vi "1ZZTEMPZZ.vi"(8 "error in":errorcluster, 9 "Message":string="Labview Stopped due to Insuficient Space", 10 "Subject":string="Labview Stopped due to Insuficient Space", 11 "Recipients":string="jtp246@cornell.edu") -> (0 "error out":errorcluster)   [LabVIEW 2023]
doc: "<p>Creates and sends an email according to the settings you specify in the configuration dialog box.</p>\n--------------------\n\nThis Express VI is configured as follows:\n\nThis VI can be used to programmatically send emails"
uses:
  GUI2.vi
  <vilib>/smtpClient/LabVIEWSMTPClient.lvlib
panel:
  in  "Require Log-in":bool=TRUE
  in  "Sender's Email Address":string="jtp246@cornell.edu"
  in  "Use Secure Connection (TLS\\SSL":bool=TRUE
  in  "Password":string="yult ybhd eril bmmg"
  in  "Port":u16=25
  in  "Username":string="b56ainvertedmicroscope@gmail.com"
  in  "Outgoing Mail Server (SMTP)":string="smtp.gmail.com"
  # "Refer to the LabVIEW Help,\navailable by selecting\nHelp>Search the\nLabVIEW Help, for\ninformation about\ndesigning \"source VIs\".\n(Include quotes)"
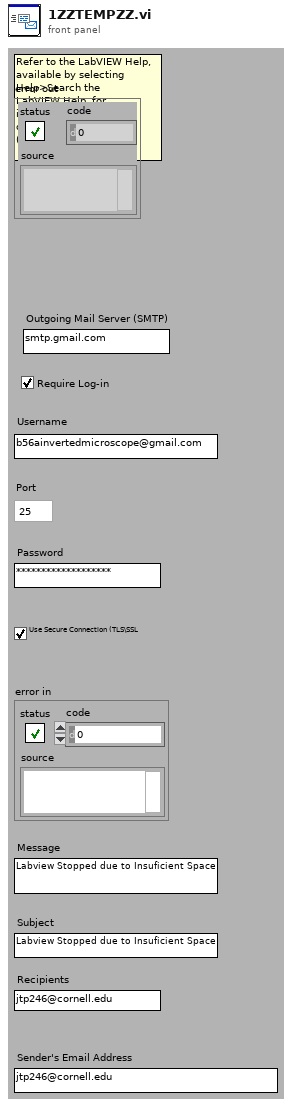
[diagram p1: front panel]
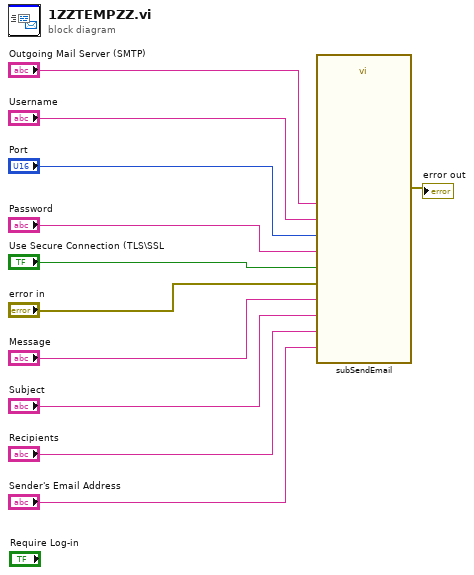
[diagram p0: block diagram]
diagram:
  n1 = call <vilib>:"subSendEmail.vi"("Sender's Email Address"="Sender's Email Address", "Recipients"="Recipients", "Subject"="Subject", "Message"="Message", "error in (no error)"="error in", "Use Secure Connection (TLS\\SSL"="Use Secure Connection (TLS\\SSL", "Password"="Password", "Port"="Port", "Username"="Username", "Outgoing Mail Server (SMTP)"="Outgoing Mail Server (SMTP)") -> ("error out"=→"error out":errorcluster)  [unwired: 9 in]
